vi "Application Aborted MHLC.vi"(8 "error in (no error)":errorcluster, 10 "Data in":variant, 11 "AppMgr in":refnum<class "Application Manager.lvclass">) -> (0 "error out":errorcluster, 3 "AppMgr out":refnum<class "Application Manager.lvclass">)   [LabVIEW 2017, in "Application Manager.lvclass"]
doc: "Workers application was pre-maturely aborted. Update status of all Workers in corresponding Workers applicaiton in tree."
uses:
  Application Manager.lvclass
  C:/Program Files (x86)/National Instruments/LabVIEW 2017/vi.lib/addons/_Workers/Library/Classes/Worker/Worker.lvclass
  <vilib>/addons/_Workers/Library/Classes/Worker/Worker.lvclass/Worker.ctl
  <vilib>/addons/_Workers/Library/Classes/Message/Message.lvclass/Message.ctl
  Application Manager.lvclass/Application Manager.ctl
  <vilib>/addons/_Workers/Library/Classes/Worker/Read Message.vi
  <vilib>/addons/_Workers/Library/Classes/Message/Read Sender WID.vi
  Common VIs/DC Name to DC_UID.vi
  <vilib>/Utility/error.llb/Error Cluster From Error Code.vi
  <vilib>/ErrorRing/Error Ring.xnode
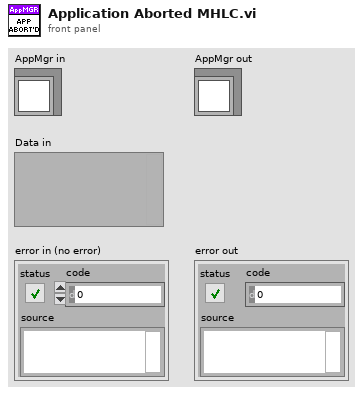
[diagram p1: front panel]
types:
  T1 = typedef "DC_UID.ctl" = string
  T2 = typedef "Application Manager.lvclass/Debug Client Data.ctl" = cluster{"DC_UID":T1, "IP Address":string, "Worker Data":T3[], "Connected":bool}
  T3 = typedef "Application Manager.lvclass/Worker Data.ctl" = cluster{"ID":string, "VI Ref":refnum<vi>, "VI Path":path, "CloneID":string, "Type":T4, "Worker Status":string}
  T4 = typedef "Workers.lvlib/Worker.lvclass/Worker Type.ctl" = enum16{"SL", "DL"}
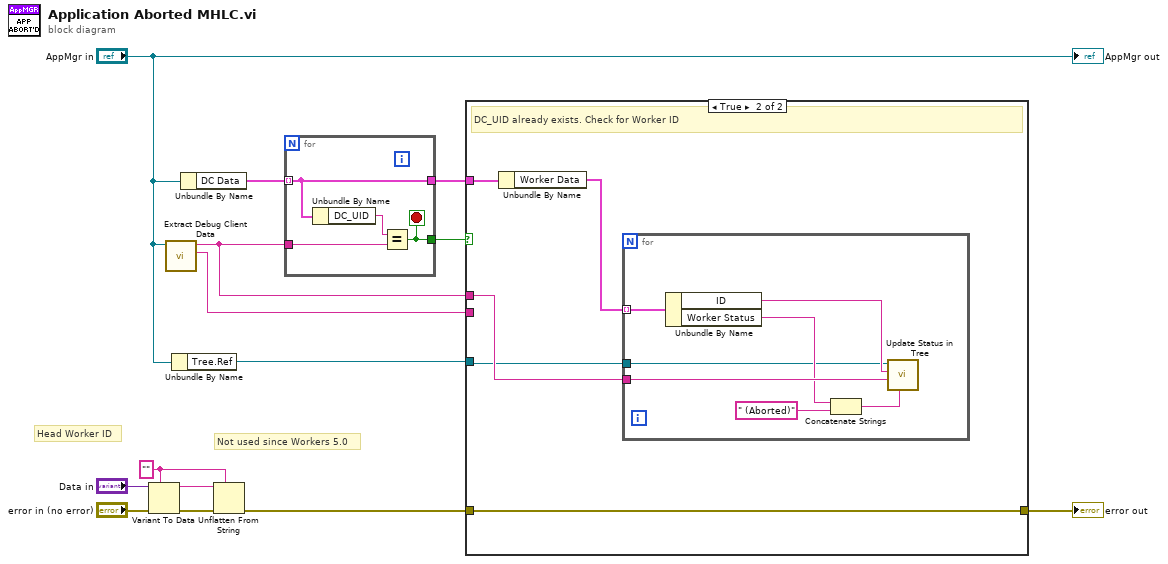
[diagram p0: block diagram]
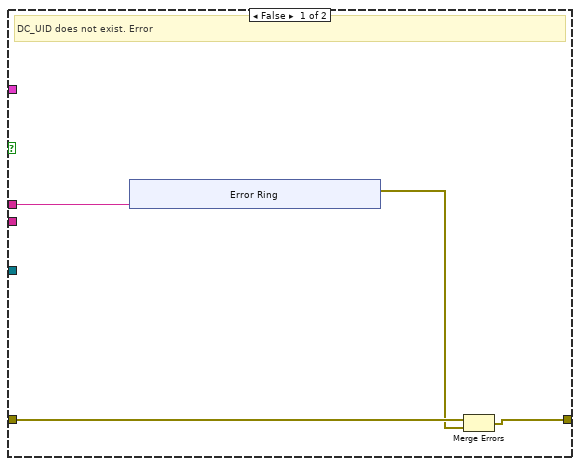
[diagram p2: hidden frame]
diagram:
  w3 = ""
  # "Not used since Workers 5.0"
  # "Head Worker ID"
  n1 = Variant To Data(error in="error in (no error)", type=w3, Variant="Data in") -> (data=w13:string, error out=w14:errorcluster)
  n2 = call "Extract Debug Client Data.vi"("AppMgr in"="AppMgr in") -> ("IP Address"=w10:string, "DC_UID"=w11:T1)  [unwired: 9 in]
  n3 = Unbundle By Name("AppMgr in") -> ("Tree.Ref"=w2:refnum<vi>)
  n4 = Unbundle By Name("AppMgr in") -> ("DC Data"=w12:T2[])
  n5 = Unflatten From String(type=w3, binary string=w13, error in (no error)=w14) -> (error out=w7:errorcluster)  [unwired: 2 in, 2 out]
  n6 = for {
    tunnel: w12 -> [w15] mode=indexing
    tunnel: w11 -> [w17]
    tunnel: [w16] -> w8
    tunnel: [w15] -> w9
    stop <- w16 stop-if-true
    n7 = Unbundle By Name(w15) -> ("DC_UID"=w18:T1)
    n8 = Equal?(x=w18, y=w17) -> (x = y?=w16:bool)
  }
  n9 = case shown="True" w8 {
    tunnel: w11 -> [w19 w31]
    tunnel: w10 -> [_ _]
    tunnel: w2 -> [_ w30]
    tunnel: w9 -> [_ w34]
    tunnel: [w21 w32] -> w6
    tunnel: w7 -> [w22 w32]
    frame False {
      # "DC_UID does not exist. Error"
      n10 = xnode "Error Ring"("parameter 0"=w19) -> ("error out"=w20:errorcluster)
      n11 = Merge Errors(w22, w20) -> (w21:errorcluster)
    }
    frame True {
      # "DC_UID already exists. Check for Worker ID"
      n12 = Unbundle By Name(w34) -> ("Worker Data"=w33:T3[])
      n13 = for {
        tunnel: w33 -> [w41] mode=indexing
        tunnel: w31 -> [w40]
        tunnel: w30 -> [w35]
        n14 = Unbundle By Name(w41) -> ("ID"=w39:string, "Worker Status"=w37:string)
        n15 = Concatenate Strings(w37, " (Aborted)" ("string")) -> (w36:string)
        n16 = call "Update Status in Tree.vi"("Worker Status"=w36, "DC_UID"=w40, "WID"=w39, "Tree Ref"=w35) -> ()  [unwired: 7 in, 1 out]
      }
    }
  }
  "error out" <- w6
  "AppMgr out" <- "AppMgr in"
